vi "采配水流程与超标留样交互.vi"(11 "参数":T1) -> ()   [LabVIEW 2016, in "PLC.lvlib"]
uses:
  PLC.lvlib
panel:
  out "输出数组":cluster{"参数名":string, "浓度":dbl}[](array[cluster])
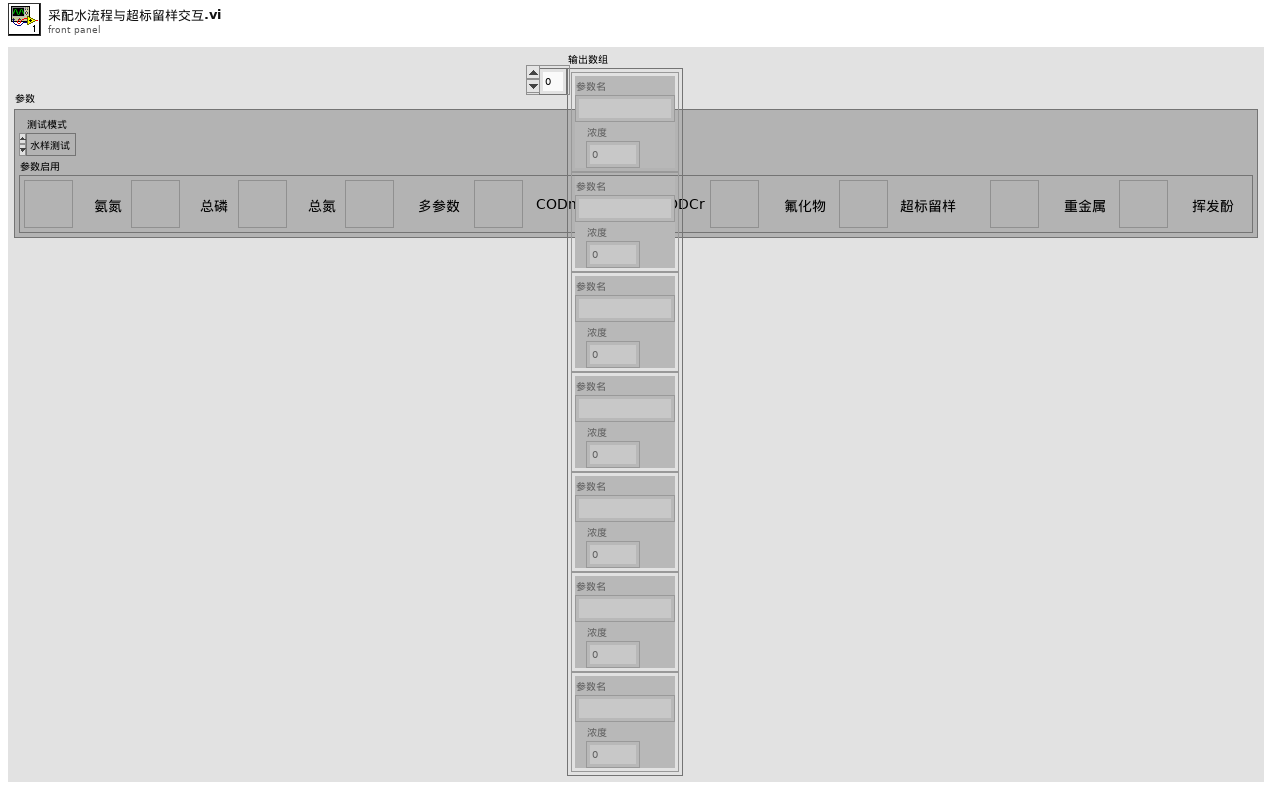
[diagram p1: front panel]
types:
  T1 = typedef "参数.ctl" = cluster{"测试模式":enum16{"水样测试", "平行样测试", "集成干预测试", "加标回收"}, "参数启用":T2}
  T2 = typedef "启动参数.ctl" = cluster{"氨氮":bool, "总磷":bool, "总氮":bool, "多参数":bool, "CODmn":bool, "CODCr":bool, "氟化物":bool, "超标留样":bool, "重金属":bool, "挥发酚":bool}
  T3 = cluster{"水样数据时间":timestamp, "水温":dbl, "pH":dbl, "DO":dbl, "DOper":dbl, "电导率":dbl, "ORP":dbl, "浊度":dbl, "叶绿素a":dbl, "藻密度":dbl, "COD":dbl, "DO2":dbl, "DO2per":dbl, "氯化物":dbl, "氨氮":dbl, "水中油":dbl}
  T4 = cluster{"温度测量值":sgl, "测量值":sgl, "温度偏移修正值":sgl, "信号值":sgl, "数据标识":string}
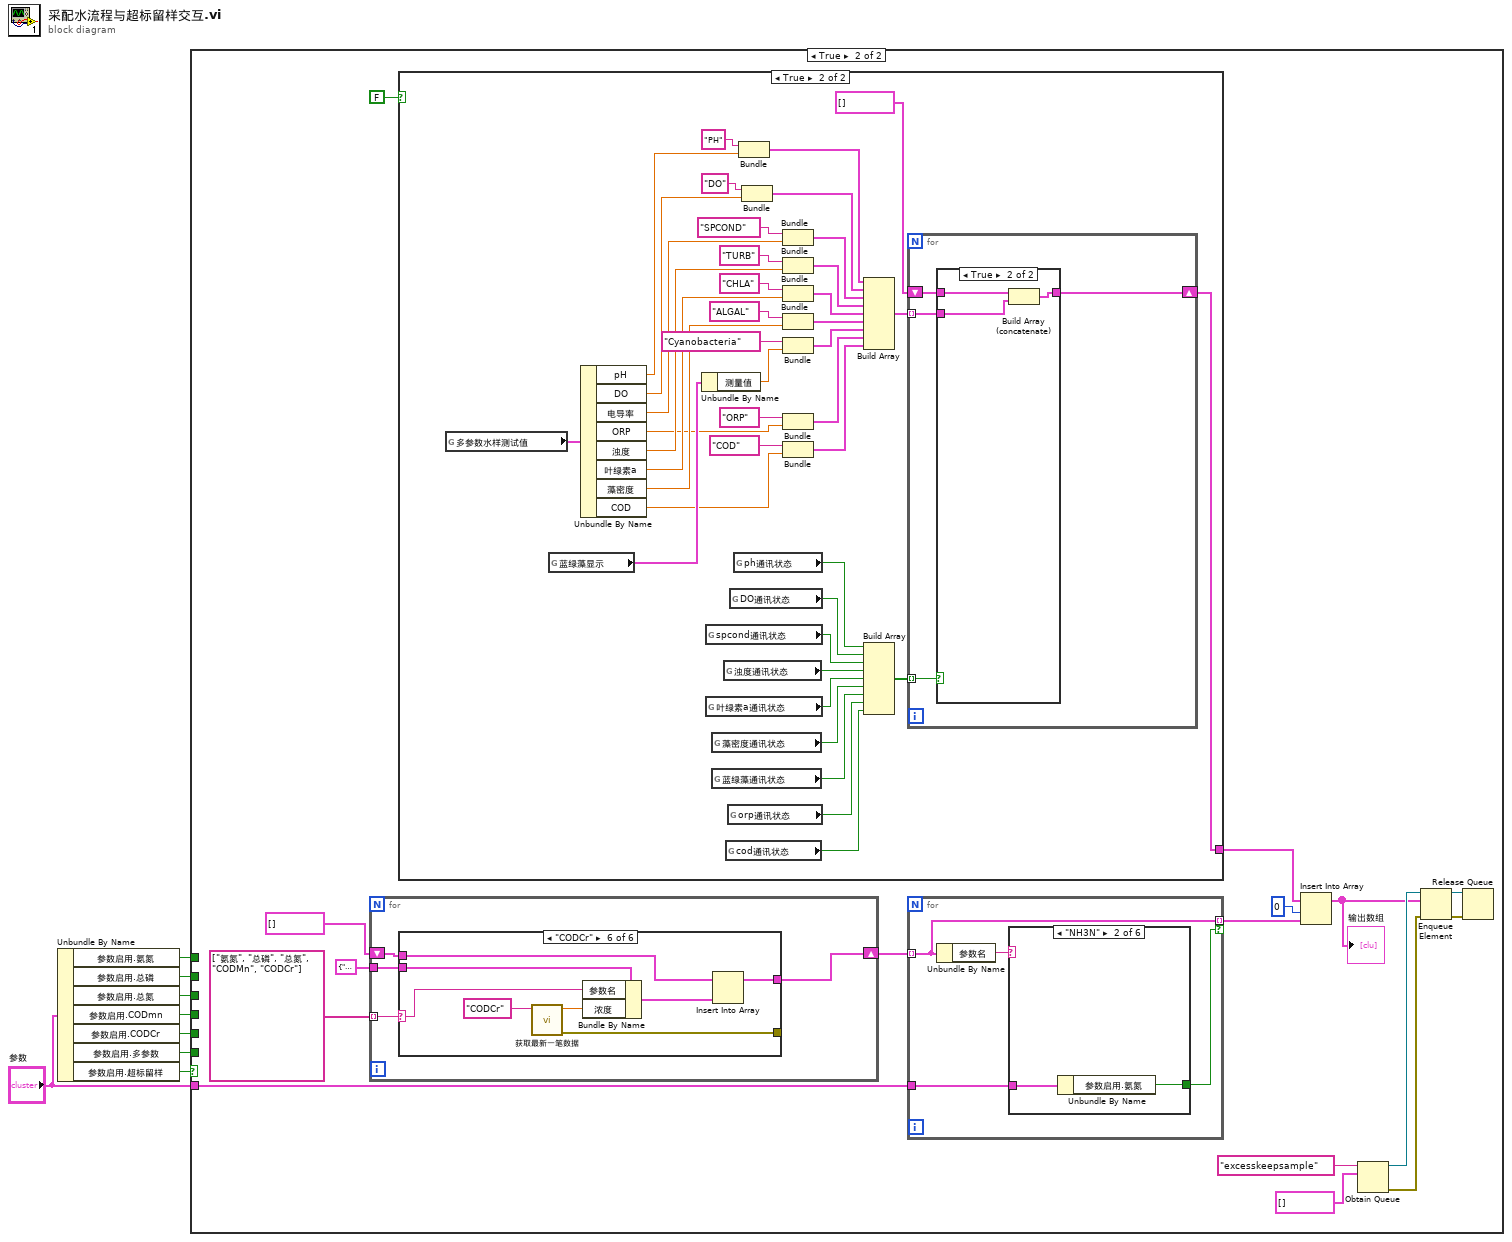
[diagram p0: block diagram]
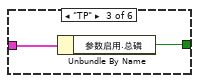
[diagram p4: hidden frame]
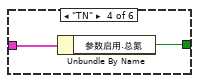
[diagram p5: hidden frame]
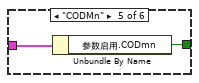
[diagram p6: hidden frame]
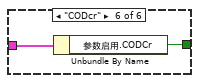
[diagram p7: hidden frame]
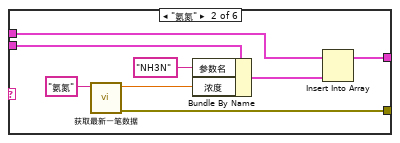
[diagram p9: hidden frame]
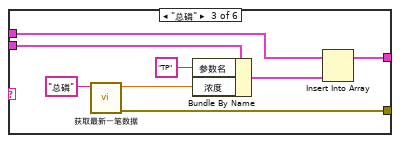
[diagram p10: hidden frame]
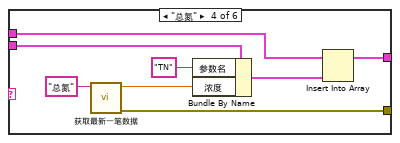
[diagram p11: hidden frame]
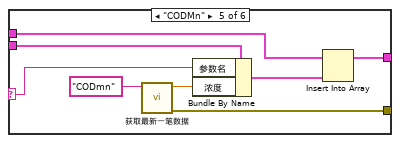
[diagram p12: hidden frame]
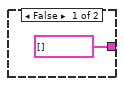
[diagram p13: hidden frame]
diagram:
  n1 = Unbundle By Name("参数") -> ("参数启用.氨氮"=w3:bool, "参数启用.总磷"=w4:bool, "参数启用.总氮"=w5:bool, "参数启用.CODmn"=w6:bool, "参数启用.CODCr"=w7:bool, "参数启用.多参数"=w8:bool, "参数启用.超标留样"=w2:bool)
  n2 = case shown="True" w2 {
    tunnel: w8 -> [_ _]
    tunnel: w7 -> [_ _]
    tunnel: w6 -> [_ _]
    tunnel: w5 -> [_ _]
    tunnel: w4 -> [_ _]
    tunnel: w3 -> [_ _]
    tunnel: "参数" -> [_ w10]
    frame False {
    }
    frame True {
      n3 = for {
        tunnel: string[] ["氨氮", "总磷", "总氮", "CODMn", "CODCr"] -> [w42] mode=indexing
        shift-right: [w39] -> w14
        shift-left: cluster{"参数名":string, "浓度":sgl}[] [] -> [w40]
        tunnel: cluster{"参数名":string, "浓度":sgl} {"参数名"="", "浓度"=0.0} ("cluster") -> [w41]
        n4 = case shown="\"CODCr\"" w42 {
          selector: w42 -> [_ _ _ _ w72 w77]
          tunnel: [_ w51 w59 w67 w75 w83] -> _
          tunnel: w41 -> [_ w44 w54 w60 w68 w78]
          tunnel: w40 -> [w43 w47 w55 w63 w71 w80]
          tunnel: [w43 w46 w53 w62 w70 w79] -> w39
          frame Default {
          }
          frame "氨氮" {
            n5 = call "获取最新一笔数据.vi"("table"="氨氮") -> ("错误输出"=w51:errorcluster, "data"=w45:dbl)  [unwired: 8 in, 1 out]
            n6 = Bundle By Name(cluster=w44, "参数名"="NH3N", "浓度"=w45) -> (w49:cluster{"参数名":string, "浓度":sgl})
            n7 = Insert Into Array(array=w47, new element=w49) -> (w46:cluster{"参数名":string, "浓度":sgl}[])  [unwired: 1 in]
          }
          frame "总磷" {
            n8 = call "获取最新一笔数据.vi"("table"="总磷") -> ("错误输出"=w59:errorcluster, "data"=w52:dbl)  [unwired: 8 in, 1 out]
            n9 = Bundle By Name(cluster=w54, "参数名"="TP", "浓度"=w52) -> (w57:cluster{"参数名":string, "浓度":sgl})
            n10 = Insert Into Array(array=w55, new element=w57) -> (w53:cluster{"参数名":string, "浓度":sgl}[])  [unwired: 1 in]
          }
          frame "总氮" {
            n11 = call "获取最新一笔数据.vi"("table"="总氮") -> ("错误输出"=w67:errorcluster, "data"=w61:dbl)  [unwired: 8 in, 1 out]
            n12 = Bundle By Name(cluster=w60, "参数名"="TN", "浓度"=w61) -> (w65:cluster{"参数名":string, "浓度":sgl})
            n13 = Insert Into Array(array=w63, new element=w65) -> (w62:cluster{"参数名":string, "浓度":sgl}[])  [unwired: 1 in]
          }
          frame "CODMn" {
            n14 = call "获取最新一笔数据.vi"("table"="CODmn") -> ("错误输出"=w75:errorcluster, "data"=w69:dbl)  [unwired: 8 in, 1 out]
            n15 = Bundle By Name(cluster=w68, "参数名"=w72, "浓度"=w69) -> (w73:cluster{"参数名":string, "浓度":sgl})
            n16 = Insert Into Array(array=w71, new element=w73) -> (w70:cluster{"参数名":string, "浓度":sgl}[])  [unwired: 1 in]
          }
          frame "CODCr" {
            n17 = call "获取最新一笔数据.vi"("table"="CODCr") -> ("错误输出"=w83:errorcluster, "data"=w76:dbl)  [unwired: 8 in, 1 out]
            n18 = Bundle By Name(cluster=w78, "参数名"=w77, "浓度"=w76) -> (w81:cluster{"参数名":string, "浓度":sgl})
            n19 = Insert Into Array(array=w80, new element=w81) -> (w79:cluster{"参数名":string, "浓度":sgl}[])  [unwired: 1 in]
          }
        }
      }
      n20 = case shown="True" FALSE {
        tunnel: [cluster{"参数名":string, "浓度":dbl}[] [] w94] -> w24
        frame False {
        }
        frame True {
          n21 = global read "多参数全局变量.vi" "多参数水样测试值"() -> (w93:T3)
          n22 = global read "多参数全局变量.vi" "蓝绿藻显示"() -> (w126:T4)
          n23 = Unbundle By Name(w93) -> ("pH"=w92:dbl, "DO"=w91:dbl, "电导率"=w90:dbl, "ORP"=w86:dbl, "浊度"=w89:dbl, "叶绿素a"=w88:dbl, "藻密度"=w87:dbl, "COD"=w85:dbl)
          n24 = Unbundle By Name(w126) -> ("测量值"=w100:sgl)
          n25 = global read "多参数全局变量.vi" "spcond通讯状态"() -> (w123:bool)
          n26 = global read "多参数全局变量.vi" "叶绿素a通讯状态"() -> (w121:bool)
          n27 = global read "多参数全局变量.vi" "藻密度通讯状态"() -> (w120:bool)
          n28 = global read "多参数全局变量.vi" "蓝绿藻通讯状态"() -> (w119:bool)
          n29 = global read "多参数全局变量.vi" "浊度通讯状态"() -> (w122:bool)
          n30 = global read "多参数全局变量.vi" "cod通讯状态"() -> (w117:bool)
          n31 = global read "多参数全局变量.vi" "orp通讯状态"() -> (w118:bool)
          n32 = global read "多参数全局变量.vi" "DO通讯状态"() -> (w124:bool)
          n33 = global read "多参数全局变量.vi" "ph通讯状态"() -> (w125:bool)
          n34 = Bundle("PH", "pH"=w92) -> (w114:cluster{string, "pH":dbl})  [unwired: 1 in]
          n35 = Bundle("DO", "DO"=w91) -> (w112:cluster{string, "DO":dbl})  [unwired: 1 in]
          n36 = Bundle("SPCOND", "电导率"=w90) -> (w110:cluster{string, "电导率":dbl})  [unwired: 1 in]
          n37 = Bundle("TURB", "浊度"=w89) -> (w108:cluster{string, "浊度":dbl})  [unwired: 1 in]
          n38 = Bundle("CHLA", "叶绿素a"=w88) -> (w105:cluster{string, "叶绿素a":dbl})  [unwired: 1 in]
          n39 = Bundle("ALGAL", "藻密度"=w87) -> (w104:cluster{string, "藻密度":dbl})  [unwired: 1 in]
          n40 = Bundle("Cyanobacteria", "测量值"=w100) -> (w99:cluster{string, "测量值":sgl})  [unwired: 1 in]
          n41 = Bundle("ORP", "ORP"=w86) -> (w98:cluster{string, "ORP":dbl})  [unwired: 1 in]
          n42 = Bundle("COD", "COD"=w85) -> (w97:cluster{string, "COD":dbl})  [unwired: 1 in]
          n43 = Build Array(w114, w112, w110, w108, w105, w104, w99, w98, w97) -> (w96:cluster{string, "COD":dbl}[])
          n44 = Build Array(w125, w124, w123, w122, w121, w120, w119, w118, w117) -> (w95:bool[])
          n45 = for {
            shift-right: [w129] -> w94
            shift-left: cluster{"参数名":string, "浓度":dbl}[] [] -> [w130]
            tunnel: w96 -> [w128] mode=indexing
            tunnel: w95 -> [w127] mode=indexing
            n46 = case shown="True" w127 {
              tunnel: w130 -> [w131 w134]
              tunnel: [w131 w133] -> w129
              tunnel: w128 -> [_ w132]
              frame False {
              }
              frame True {
                n47 = Build Array (concatenate)(w134, w132) -> (w133:cluster{"参数名":string, "COD":dbl}[])
              }
            }
          }
        }
      }
      n48 = for {
        tunnel: w14 -> [w27] mode=indexing
        tunnel: [w27] -> w9 mode=indexing if=w25
        tunnel: w10 -> [w26]
        n49 = Unbundle By Name(w27) -> ("参数名"=w28:string)
        n50 = case shown="\"NH3N\"" w28 {
          tunnel: w26 -> [_ w30 w32 w34 w36 w38]
          tunnel: [_ w29 w31 w33 w35 w37] -> w25
          frame "False", Default {
          }
          frame "NH3N" {
            n51 = Unbundle By Name(w30) -> ("参数启用.氨氮"=w29:bool)
          }
          frame "TP" {
            n52 = Unbundle By Name(w32) -> ("参数启用.总磷"=w31:bool)
          }
          frame "TN" {
            n53 = Unbundle By Name(w34) -> ("参数启用.总氮"=w33:bool)
          }
          frame "CODMn" {
            n54 = Unbundle By Name(w36) -> ("参数启用.CODmn"=w35:bool)
          }
          frame "CODcr" {
            n55 = Unbundle By Name(w38) -> ("参数启用.CODCr"=w37:bool)
          }
        }
      }
      n56 = Insert Into Array(array=w24, index=0 ("索引"), new element=w9) -> (w16:cluster{"参数名":string, "浓度":dbl}[])
      "输出数组" <- w16
      n57 = Obtain Queue(name (unnamed)="excesskeepsample" ("名称（未命名）"), element data type=cluster{"参数名":string, "浓度":dbl}[] []) -> (queue out=w20:refnum<queue>, error out=w19:errorcluster)  [unwired: 3 in, 1 out]
      n58 = Enqueue Element(queue=w20, element=w16, error in (no error)=w19) -> (queue out=w18:refnum<queue>, error out=w17:errorcluster)  [unwired: 1 in, 1 out]
      n59 = Release Queue(queue=w18, error in (no error)=w17) -> ()  [unwired: 1 in, 3 out]
    }
  }
